vi "3.3.vi"() -> ()   [LabVIEW 2017]
panel:
  in  "偏移量3":dbl
  in  "剩余 2":dbl
  out "数值":dbl
  out "字符串 2":string
  out "字符串 1":string
  in  "长度剩余":dbl
  in  "偏移量 2":dbl
  in  "字符串":string
  in  "偏移量1":dbl
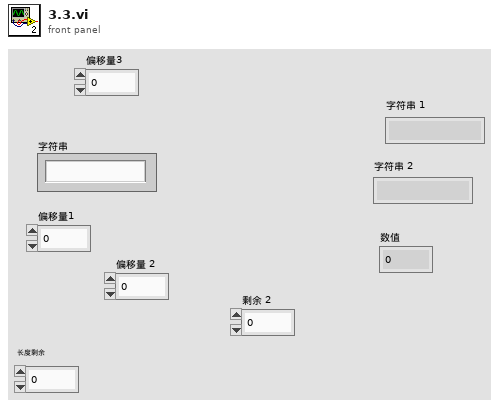
[diagram p1: front panel]
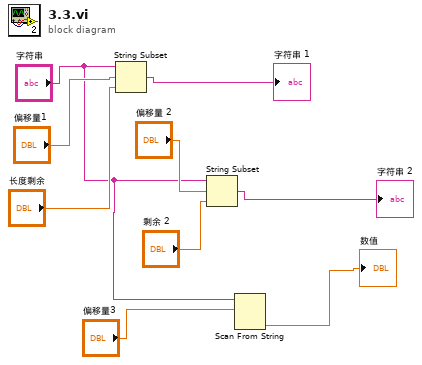
[diagram p0: block diagram]
diagram:
  n1 = String Subset(string="字符串", offset (0)="偏移量1", length (rest)="长度剩余") -> (substring=→"字符串 1":string)
  n2 = String Subset(string="字符串", offset (0)="偏移量 2", length (rest)="剩余 2") -> (substring=→"字符串 2":string)
  n3 = Scan From String(input string="字符串", initial scan location="偏移量3") -> (output 1=→"数值":dbl)  [unwired: 3 in, 3 out]
